vi "Process Session Exit Code.vi"(8 "error in (no error)":errorcluster, 11 "session ID in":i32 format="%.0x") -> (0 "error out":errorcluster, 2 "exit code":u32, 3 "session ID out":i32 format="%.0x")   [LabVIEW 2013]
uses:
  ProcessSession.dll
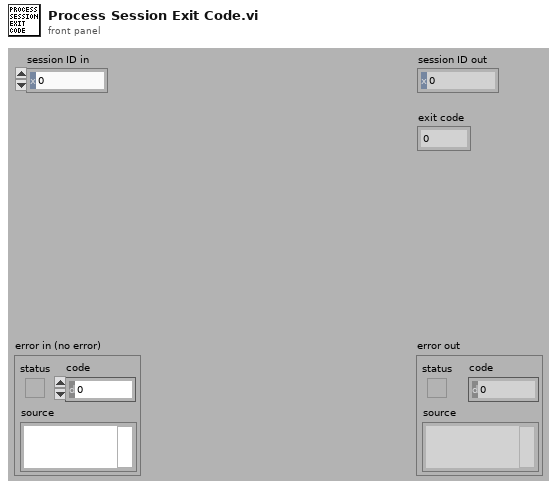
[diagram p1: front panel]
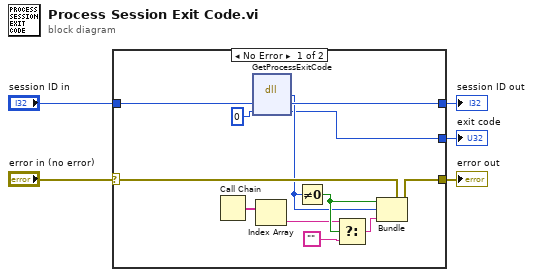
[diagram p0: block diagram]
diagram:
  n1 = case shown="No Error" "error in (no error)" {
    selector: "error in (no error)" -> [w17 w19]
    tunnel: [w10 w18] -> w5
    tunnel: [w13 w19] -> w3
    tunnel: [w8 _] -> w2
    tunnel: "session ID in" -> [w6 w18]
    frame No Error {
      n2 = Call Chain() -> (call chain=w12:string[])
      n3 = dll-call lib="C:/Users/inghoshr/Documents/LabVIEW Data/SmoketestVMVi/Process Session/ProcessSession.dll" fn="GetProcessExitCode"("session"=w6, "exitCode"=u32 0 ("stillRunning")) -> (w9:i32, "session"=w10:i32, "exitCode"=w8:u32)  [unwired: 3 in, 2 out]
      n4 = Index Array(array=w12) -> (element=w11:string)  [unwired: 1 in]
      n5 = Not Equal To 0?(x=w9) -> (x != 0?=w16:bool)
      n6 = Select(t=w11, s=w16, f="") -> (s? t:f=w14:string)
      n7 = Bundle(cluster=w17, "status"=w16, "code"=w9, "source"=w14) -> (w13:errorcluster)
    }
    frame Error {
    }
  }
  "session ID out" <- w5
  "error out" <- w3
  "exit code" <- w2
